vi "mongo test.vi"() -> ()   [LabVIEW 2013]
panel:
  out "error out 2":errorcluster
  out "connection ID":refnum<k5>
  out "error out":errorcluster
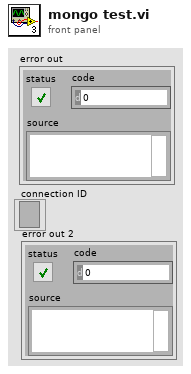
[diagram p1: front panel]
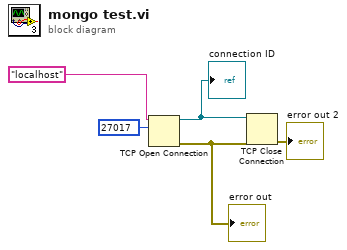
[diagram p0: block diagram]
diagram:
  n1 = TCP Open Connection(address="localhost", remote port or service name=u16 27017) -> (connection ID=w2:refnum<k5>, error out=w3:errorcluster)  [unwired: 3 in]
  "error out" <- w3
  "connection ID" <- w2
  n2 = TCP Close Connection(connection ID=w2, error in (no error)=w3) -> (error out=→"error out 2":errorcluster)  [unwired: 1 in, 1 out]
